vi "Teleop.vi"(10 "Match Info":T1={"Autonomous Elapsed Seconds"=0.0, "TeleOp Elapsed Seconds"=0.0, "Disabled Elapsed Seconds"=0.0, "Visited Autonomous"=FALSE, "Visited TeleOp"=FALSE, "Visited Disabled"=FALSE, "Autonomous Settings"={"Autonomous Style"=enum."Independent", "VI Refnum"=refnum}}, 11 "Call Context":T2) -> ()   [LabVIEW 2015]
doc: "This VI is called for each TeleOp packet received from the DS where the robot is not disabled. It is often used to read from the joysticks and update I/O or to update setpoints for timed control loops. It should complete and return within 20 milliseconds or it may miss DS packets."
uses:
  <vilib>/Rock Robotics/WPI/DriverStation/WPI_DriverStationDerivedRobotMode.ctl
  <vilib>/Rock Robotics/WPI/DriverStation/WPI_DriverStationMatch Info.ctl
  <vilib>/Rock Robotics/WPI/Utilities/WPI_GetSetVariantRefNum.vi
  <vilib>/addons/control/pid/pid.llb/PID Output Rate Limiter (DBL).vi
  <vilib>/addons/control/pid/NI_PID_pid.lvlib
panel:
  out "Right Chart":dbl(graph)
  out "Left Chart":dbl(graph)
  in  "dt (s)":dbl=2.0 format="%.2f"
  in  "output rate (EGU/min)":dbl=25.0 format="%.2f"
  in  "initial output":dbl format="%.2f"
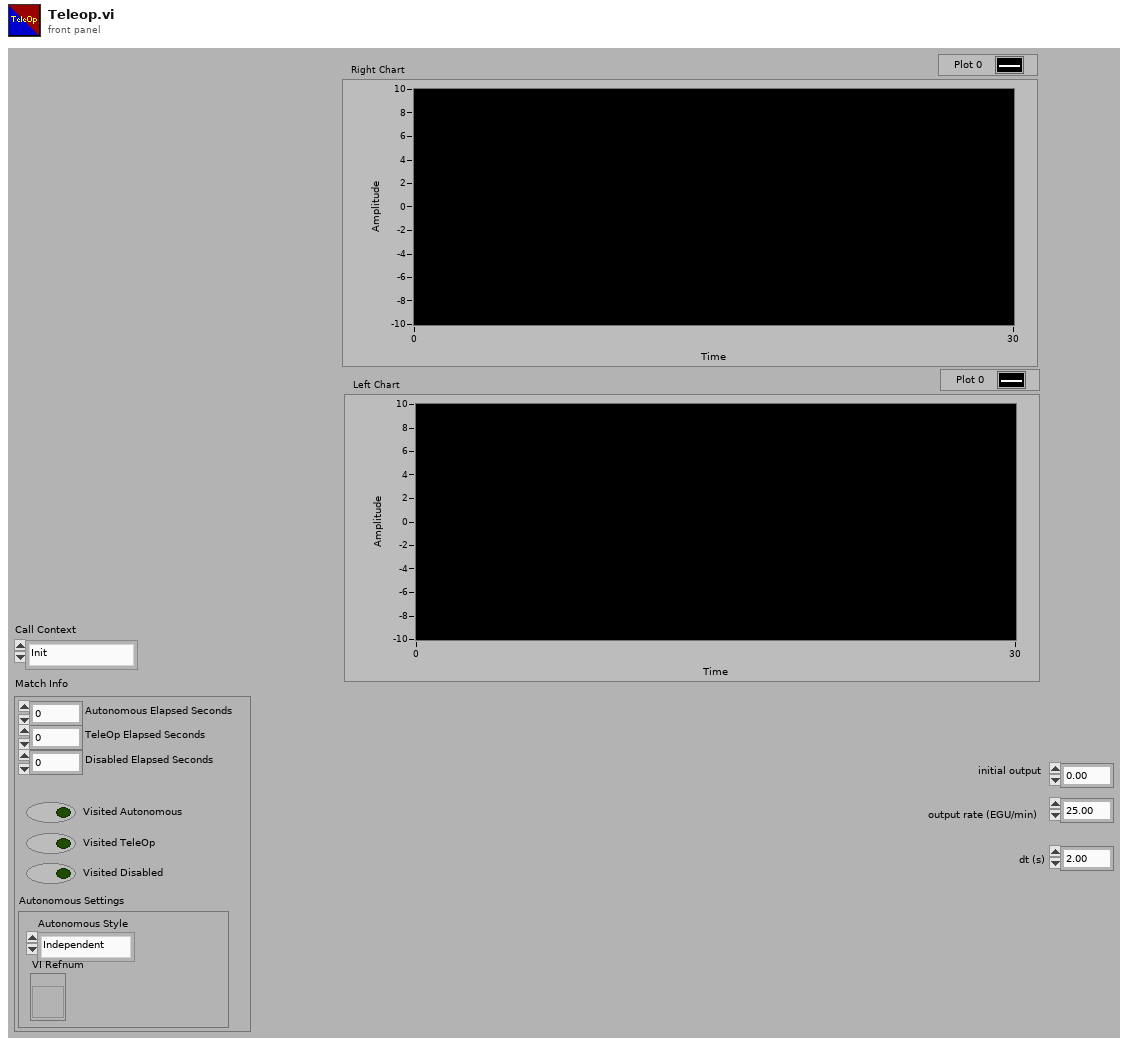
[diagram p1: front panel]
types:
  T1 = typedef "WPI_DriverStationMatch Info.ctl" = cluster{"Autonomous Elapsed Seconds":dbl, "TeleOp Elapsed Seconds":dbl, "Disabled Elapsed Seconds":dbl, "Visited Autonomous":bool, "Visited TeleOp":bool, "Visited Disabled":bool, "Autonomous Settings":cluster{"Autonomous Style":enum16{"Iterative", "Independent"}, "VI Refnum":refnum<vi>}}
  T2 = typedef "WPI_DriverStationDerivedRobotMode.ctl" = enum16{"Init", "Execute", "Stop"}
  T3 = typedef "WPI_JoystickDevRef.ctl" = cluster{"Device":T4}
  T4 = typedef "WPI_JoystickDeviceEnum.ctl" = enum16{"USB 0", "USB 1", "USB 2", "USB 3", "USB 4", "USB 5"}
  T5 = typedef "WPI_RobotDriveDevRef.ctl" = cluster{"DevStatus":errorcluster, "Motors[]":T6[], "Square Inputs":bool, "Max Output":dbl}
  T6 = typedef "WPI_MotorControlDeviceRef.ctl" = cluster{"DeviceStatus":errorcluster, "Type":T7, "PWM":cluster{"PWM Channel":T8, "DeadBand":T9}, "CAN":cluster{"Device Number":u8, "Control Mode":T10, "Semaphore":T11, "Max Vout":dbl, "TalonSRX Control Mode":T12}, "Invert":bool}
  T7 = typedef "WPI_MotorControlType.ctl" = enum16{"PWM", "CAN", "CANTalonSRX"}
  T8 = typedef "FPGA_DIOPWMChannel.ctl" = enum8{"PWM 0", "PWM 1", "PWM 2", "PWM 3", "PWM 4", "PWM 5", "PWM 6", "PWM 7", "PWM 8", "PWM 9", "PWM MXP 0", "PWM MXP 1", "PWM MXP 2", "PWM MXP 3", "PWM MXP 4", "PWM MXP 5", "PWM MXP 6", "PWM MXP 7", "PWM MXP 8", "PWM MXP 9", "Invalid"}
  T9 = typedef "WPI_PWMDeadband.ctl" = cluster{"Name":string, "maxPositivePwm":i32, "minPositivePwm":i32, "centerPwm":i32, "maxNegativePwm":i32, "minNegativePwm":i32, "angularRange":u16}
  T10 = typedef "WPI_CANJaguar_ControlMode.ctl" = enum8{"Percent VBus", "Current", "Speed", "Position", "Voltage"}
  T11 = typedef "Semaphore RefNum" = refnum<k1>
  T12 = typedef "WPI_CANTalonSRX_APIControlMode.ctl" = enum8{"Percent VBus", "Speed", "Position", "Slave", "Unchanged / Invalid", "Voltage Compensation", "Current", "Motion Profile"}
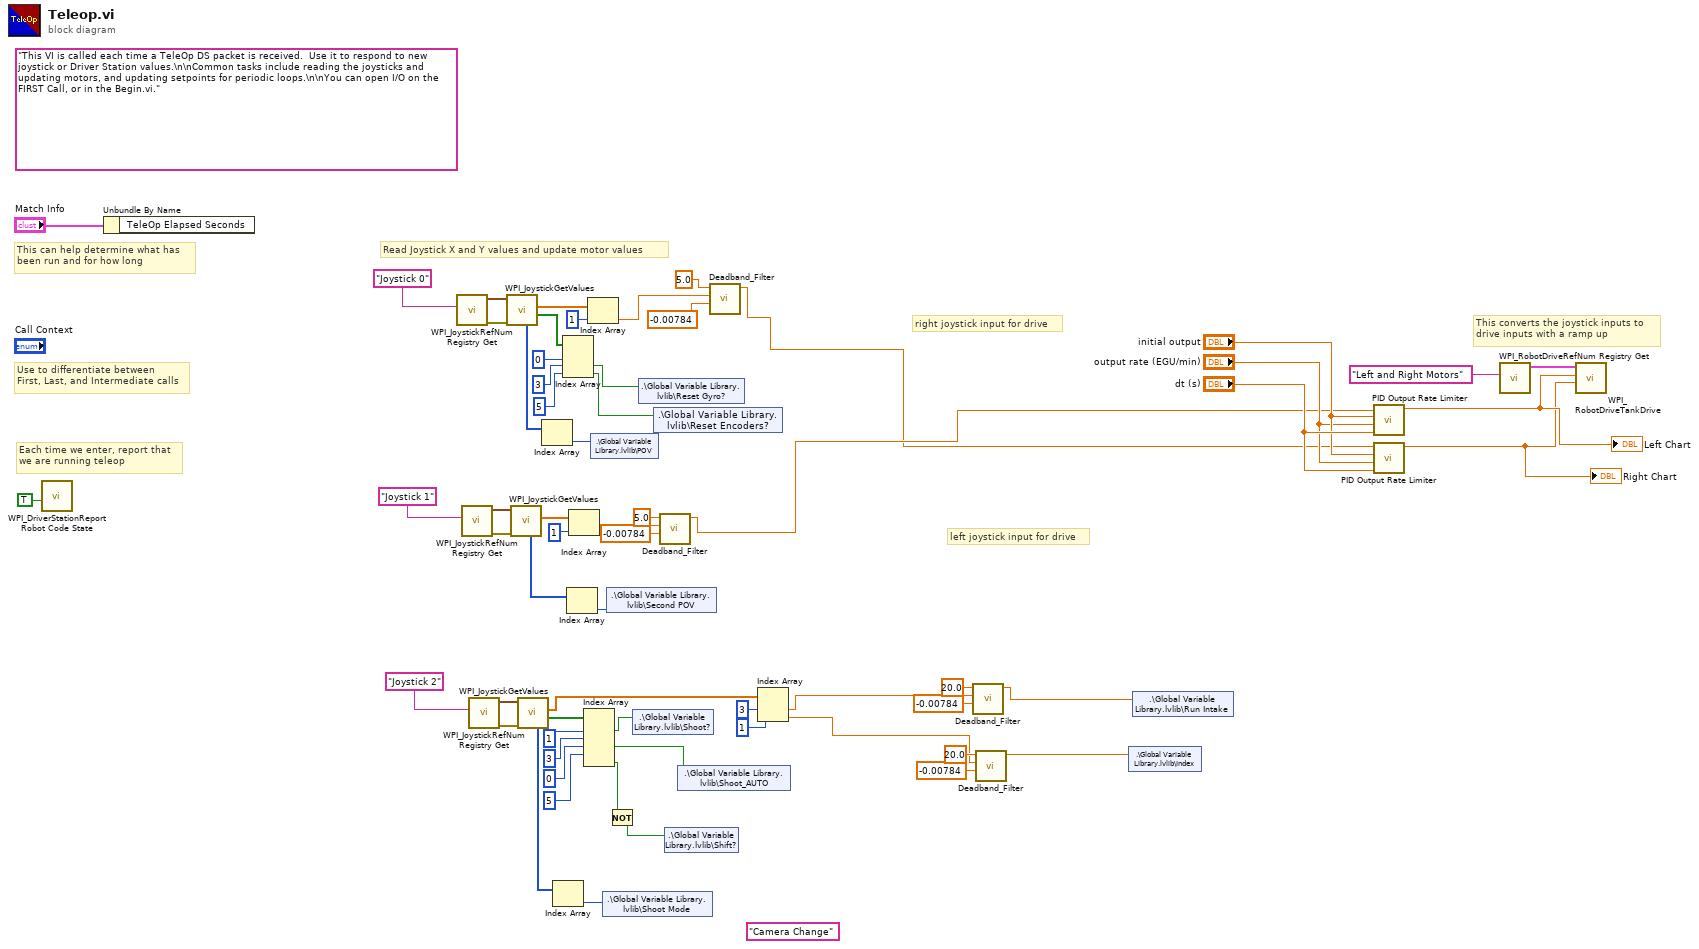
[diagram p0: block diagram]
diagram:
  (unwired) "Camera Change" ("Name")
  (unwired) "This VI is called each time a TeleOp DS packet is received.  Use it to respond to new joystick or Driver Station values.\n\nCommon tasks include reading the joysticks and updating motors, and updating setpoints for periodic loops.\n\nYou can open I/O on the FIRST Call, or in the Begin.vi."
  # "This converts the joystick inputs to\ndrive inputs with a ramp up"
  # "left joystick input for drive"
  # "right joystick input for drive"
  # "Each time we enter, report that\nwe are running teleop"
  # "Use to differentiate between\nFirst, Last, and Intermediate calls"
  # "This can help determine what has\nbeen run and for how long"
  # "Read Joystick X and Y values and update motor values"
  n1 = call <vilib>:"WPI_DriverStationReport Robot Code State.vi"("TeleOp"=TRUE ("Autonomous")) -> ()  [unwired: 10 in, 1 out]
  n2 = Unbundle By Name("Match Info") -> ()  [unwired: 1 out]
  n3 = call <vilib>:"WPI_JoystickRefNum Registry Get.vi"("refnum name"="Joystick 0") -> ("error out"=w57:errorcluster, "JoystickDevRef"=w56:T3)  [unwired: 1 in, 8 out]
  n4 = call <vilib>:"WPI_JoystickRefNum Registry Get.vi"("refnum name"="Joystick 1") -> ("error out"=w51:errorcluster, "JoystickDevRef"=w50:T3)  [unwired: 1 in, 8 out]
  n5 = call <vilib>:"WPI_JoystickRefNum Registry Get.vi"("refnum name"="Joystick 2") -> ("error out"=w48:errorcluster, "JoystickDevRef"=w47:T3)  [unwired: 1 in, 8 out]
  n6 = call <vilib>:"WPI_JoystickGetValues.vi"("error in (no error)"=w57, "JoystickDevRef"=w56) -> ("Buttons"=w54:bool[], "Axes"=w55:dbl[], "POVs"=w53:i16[])  [unwired: 5 in, 2 out]
  n7 = call <vilib>:"WPI_JoystickGetValues.vi"("error in (no error)"=w51, "JoystickDevRef"=w50) -> ("Axes"=w49:dbl[], "POVs"=w30:i16[])  [unwired: 5 in, 3 out]
  n8 = call <vilib>:"WPI_JoystickGetValues.vi"("error in (no error)"=w48, "JoystickDevRef"=w47) -> ("Buttons"=w46:bool[], "Axes"=w26:dbl[], "POVs"=w33:i16[])  [unwired: 5 in, 2 out]
  n9 = Index Array(array=w53) -> (element=w52:i16)  [unwired: 1 in]
  n10 = Index Array(array=w33) -> (element=w32:i16)  [unwired: 1 in]
  n11 = Index Array(array=w54, index #1=0 ("index"), index #2=3 ("index"), index #3=5 ("index")) -> (element #2=w31:bool, element #3=w13:bool)  [unwired: 1 out]
  n12 = Index Array(array=w30) -> (element=w29:i16)  [unwired: 1 in]
  n13 = Index Array(array=w49, index=1) -> (element=w39:dbl)
  n14 = Index Array(array=w46, index #1=1 ("index"), index #2=3 ("index"), index #3=0 ("index"), index #4=5 ("index")) -> (element #1=w45:bool, element #3=w5:bool, element #5=w2:bool)  [unwired: 1 in, 2 out]
  n15 = Index Array(array=w55, index=1) -> (element=w34:dbl)
  n16 = shared-variable ".\\Global Variable Library.lvlib\\POV"(w52) -> ()  [unwired: 1 in, 1 out]
  n17 = shared-variable ".\\Global Variable Library.lvlib\\Shoot Mode"(w32) -> ()  [unwired: 1 in, 1 out]
  n18 = shared-variable ".\\Global Variable Library.lvlib\\Second POV"(w29) -> ()  [unwired: 1 in, 1 out]
  n19 = Not(x=w2) -> (.not. x?=w1:bool)
  n20 = shared-variable ".\\Global Variable Library.lvlib\\Shoot?"(w45) -> ()  [unwired: 1 in, 1 out]
  n21 = shared-variable ".\\Global Variable Library.lvlib\\Reset Gyro?"(w31) -> ()  [unwired: 1 in, 1 out]
  n22 = shared-variable ".\\Global Variable Library.lvlib\\Reset Encoders?"(w13) -> ()  [unwired: 1 in, 1 out]
  n23 = call "Deadband_Filter.vi"("Deadband_Center"=-0.00784, "Input"=w39, "Deadband_Size(%)"=5.0) -> ("Deadbanded_Output"=w7:dbl)  [unwired: 8 in]
  n24 = shared-variable ".\\Global Variable Library.lvlib\\Shift?"(w1) -> ()  [unwired: 1 in, 1 out]
  n25 = shared-variable ".\\Global Variable Library.lvlib\\Shoot_AUTO"(w5) -> ()  [unwired: 1 in, 1 out]
  n26 = call "Deadband_Filter.vi"("Deadband_Center"=-0.00784, "Input"=w34, "Deadband_Size(%)"=5.0) -> ("Deadbanded_Output"=w6:dbl)  [unwired: 8 in]
  n27 = Index Array(array=w26, index #1=3 ("index"), index #2=1 ("index")) -> (element #1=w19:dbl, element #2=w16:dbl)
  n28 = call "Deadband_Filter.vi"("Deadband_Center"=-0.00784, "Input"=w19, "Deadband_Size(%)"=20.0) -> ("Deadbanded_Output"=w20:dbl)  [unwired: 8 in]
  n29 = call "Deadband_Filter.vi"("Deadband_Center"=-0.00784, "Input"=w16, "Deadband_Size(%)"=20.0) -> ("Deadbanded_Output"=w15:dbl)  [unwired: 8 in]
  n30 = shared-variable ".\\Global Variable Library.lvlib\\Index"(w15) -> ()  [unwired: 1 in, 1 out]
  n31 = shared-variable ".\\Global Variable Library.lvlib\\Run Intake"(w20) -> ()  [unwired: 1 in, 1 out]
  n32 = call-poly <vilib>:"PID Output Rate Limiter.vi"("dt (s)"="dt (s)", "output rate (EGU/min)"="output rate (EGU/min)", "initial output"="initial output", "input (controller output)"=w7) -> ("output"=w4:dbl)  [unwired: 4 in, 1 out]
  "Left Chart" <- w4
  n33 = call-poly <vilib>:"PID Output Rate Limiter.vi"("dt (s)"="dt (s)", "output rate (EGU/min)"="output rate (EGU/min)", "initial output"="initial output", "input (controller output)"=w6) -> ("output"=w3:dbl)  [unwired: 4 in, 1 out]
  "Right Chart" <- w3
  n34 = call <vilib>:"WPI_RobotDriveRefNum Registry Get.vi"("refnum name"="Left and Right Motors") -> ("RobotDriveDevRef"=w11:T5)  [unwired: 9 in, 1 out]
  n35 = call <vilib>:"WPI_RobotDriveTankDrive.vi"("Right axis value"=w3, "Left axis value"=w4, "RobotDriveDevRef"=w11) -> ()  [unwired: 6 in, 3 out]
